vi "Build Array Function.vi"() -> ()   [LabVIEW 2014]
panel:
  out "二维数组":i32[][](array[numeric])
  out "连接的数组":i32[](array[numeric])
  out "拼接元素":i32[](array[numeric])
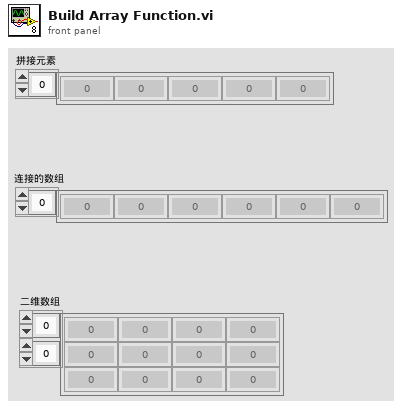
[diagram p1: front panel]
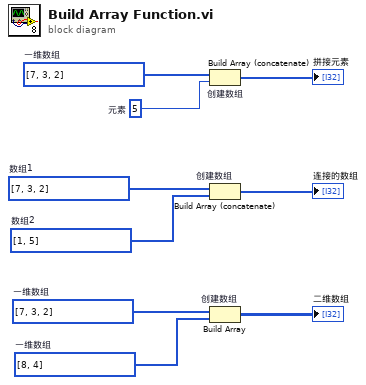
[diagram p0: block diagram]
diagram:
  w3 = i32[] [8, 4]  # 一维数组
  w2 = i32[] [7, 3, 2]  # 一维数组
  w4 = i32[] [1, 5]  # 数组2
  w5 = i32[] [7, 3, 2]  # 数组1
  w8 = 5  # 元素
  w9 = i32[] [7, 3, 2]  # 一维数组
  n1 = Build Array (concatenate) "创建数组"(w9, w8) -> (→"拼接元素":i32[])
  n2 = Build Array (concatenate) "创建数组"(w5, w4) -> (→"连接的数组":i32[])
  n3 = Build Array "创建数组"(w2, w3) -> (→"二维数组":i32[][])
